vi "1DSearch.vi"() -> ()   [LabVIEW 2023]
panel:
  out "Match 1 in 2":u64[](array[numeric])
  out "UnMatch 1 in 2":u64[](array[numeric])
  out "Match 2 in 1":u64[](array[numeric])
  out "UnMatch 2 in 1":u64[](array[numeric])
  in  "Array 2":u64[](array[numeric])
  in  "Array 1":u64[](array[numeric])
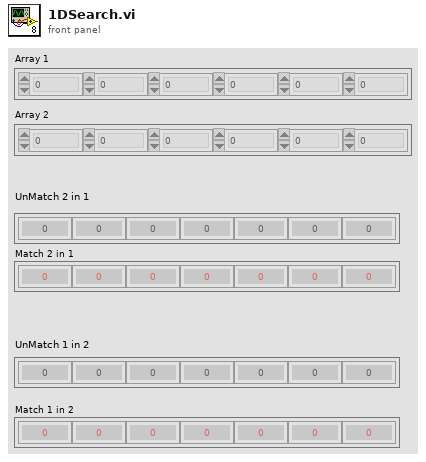
[diagram p1: front panel]
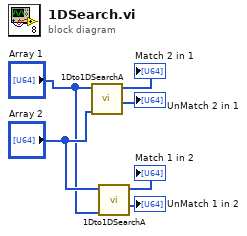
[diagram p0: block diagram]
diagram:
  n1 = call "1Dto1DSearchА.vi"("Array 2"="Array 2", "Array 1"="Array 1") -> ("UnMatch Elements"=→"UnMatch 2 in 1":u64[], "Match Elements"=→"Match 2 in 1":u64[])  [unwired: 6 in, 2 out]
  n2 = call "1Dto1DSearchА.vi"("Array 2"="Array 1", "Array 1"="Array 2") -> ("UnMatch Elements"=→"UnMatch 1 in 2":u64[], "Match Elements"=→"Match 1 in 2":u64[])  [unwired: 6 in, 2 out]
